vi "CCGetDICOMValuesFromFile.vi"(8 "error in (no error)":errorcluster, 11 "filename":string) -> (0 "error out":errorcluster, 3 "Array":string[](array[string]))   [LabVIEW 2013, in "ClearCanvasLibrary.lvlib"]
uses:
  Controls/Enum Variables.ctl
  C:/Users/Simon/SkyDrive/LabView/2013/DM2020/DICOM/ClearCanvasNewBuild/ClearCanvas.Dicom.dll
  ClearCanvasNewBuild/ClearCanvas.Dicom.dll
  ClearCanvasLibrary.lvlib
  main.lvlib
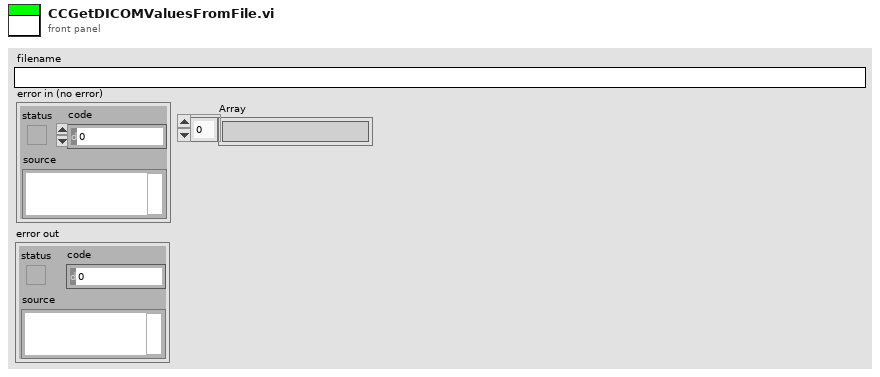
[diagram p1: front panel]
types:
  T1 = typedef "main.lvlib/Enum Variables.ctl" = enum16{"SetAcqFilter", "GetAcqFilter", "Set Filter", "Get Filter", "Set Height", "Get Height", "Set Blue Pressure", "Get Blue Pressure", "Set Red Pressure", "Get Red Pressure", "Init", "Reset Pressure", "Set Red Cursors", "Get Red Cursors", "Set Blue Cursors", "Get Blue Cursors", "Set Language", "Get Language", "Set Active Graphs", "Get ActiveGraphs", "Set Method", "Get Method", "Set Encryption", "Get Encryption", "Set ExcelVersion", "Get ExcelVersion", "Set itemTags", "Get itemTags", "Set Attributes", "Get Attributes", "Set DICOM Avail", "Get DICOM Avail", "Set DICOM Encode", "Get DICOM Encode", "Set JournalExport", "Get JournalExport", "Set Sequence", "Get Sequence", "Set DAQ Connected", "Get DAQ Connected", "Set Current Graph", "Get Current Graph", "Set General Settings", "Get Hyphenation", "Set Arm Calc Method", "Get Arm Calc Method", "Set Dicom Tags", "Get Dicom Tags"}
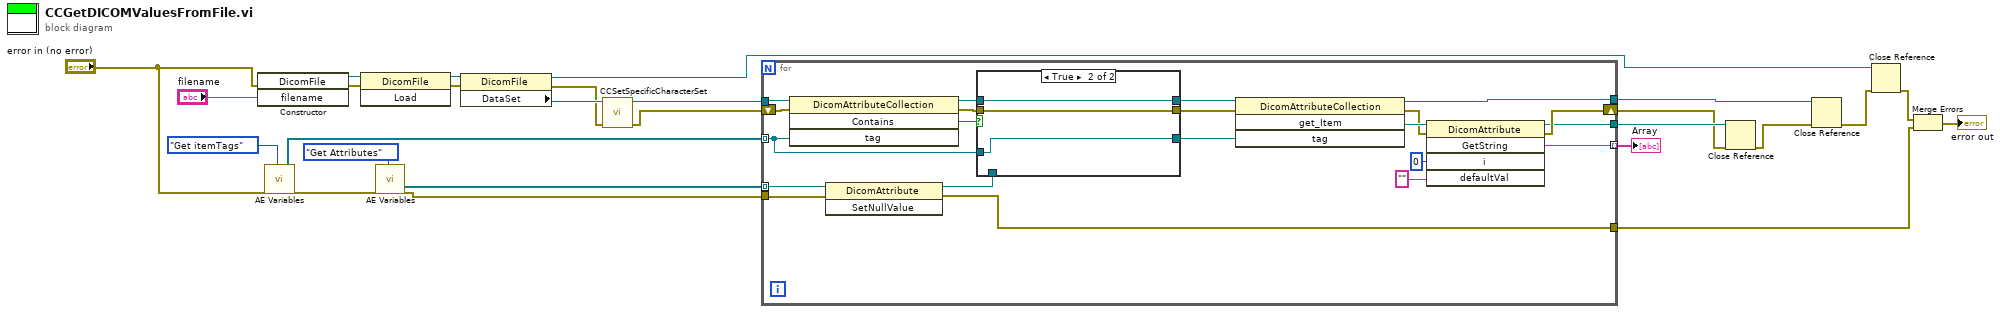
[diagram p0: block diagram]
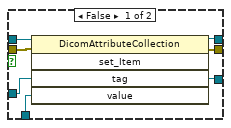
[diagram p2: hidden frame]
diagram:
  n1 = constructor class="DicomFile"(error in="error in (no error)", "filename"="filename") -> (reference out=w26:refnum<k24>, error out=w23:errorcluster)  [unwired: 2 in, 2 out]
  n2 = call "AE Variables.vi"("error in (no error)"="error in (no error)", "Action"=Enum_Variables."Get itemTags") -> ("itemTags .net"=w10:refnum<k24>[], "error out"=w9:errorcluster)  [unwired: 9 in, 7 out]
  n3 = invoke class="DicomFile" method="Load"(reference=w26, error in=w23) -> (reference out=w24:refnum<k24>, error out=w22:errorcluster)  [unwired: 1 in, 1 out]
  n4 = call "AE Variables.vi"("error in (no error)"=w9, "Action"=Enum_Variables."Get Attributes") -> (".net Array"=w7:refnum<k24>[], "error out"=w5:errorcluster)  [unwired: 9 in, 7 out]
  n5 = property class="DicomFile"(reference=w24, error in=w22) -> (reference out=w15:refnum<k24>, error out=w2:errorcluster, "DataSet"=w4:refnum<k24>)
  n6 = call "CCSetSpecificCharacterSet.vi"("error in (no error)"=w2, ".NET Refnum in"=w4) -> ("error out"=w1:errorcluster, ".NET Refnum out"=w3:refnum<k24>)  [unwired: 8 in]
  n7 = for {
    tunnel: w3 -> [w39]
    shift-right: [w42] -> w19
    shift-left: w1 -> [w38]
    tunnel: [w44] -> w21 mode=indexing
    tunnel: [w41] -> w20
    tunnel: [w40] -> w17
    tunnel: w10 -> [w33] mode=indexing
    tunnel: w7 -> [w30] mode=indexing
    tunnel: [w28] -> w6
    tunnel: w5 -> [w27]
    n8 = invoke class="DicomAttributeCollection" method="Contains"(reference=w39, error in=w38, "tag"=w33) -> (reference out=w36:refnum<k24>, error out=w34:errorcluster, "Contains"=w37:bool)  [unwired: 1 in, 1 out]
    n9 = invoke class="DicomAttribute" method="SetNullValue"(reference=w30, error in=w27) -> (reference out=w29:refnum<k24>, error out=w28:errorcluster)  [unwired: 1 in, 1 out]
    n10 = case shown="True" w37 {
      tunnel: w36 -> [w53 w56]
      tunnel: [w50 w56] -> w31
      tunnel: [w52 w55] -> w35
      tunnel: w34 -> [w51 w55]
      tunnel: w33 -> [w48 w54]
      tunnel: [w48 w54] -> w32
      tunnel: w29 -> [w49 _]
      frame False {
        n11 = invoke class="DicomAttributeCollection" method="set_Item"(reference=w53, error in=w51, "tag"=w48, "value"=w49) -> (reference out=w50:refnum<k24>, error out=w52:errorcluster)  [unwired: 1 in, 3 out]
      }
      frame True {
      }
    }
    n12 = invoke class="DicomAttributeCollection" method="get_Item"(reference=w31, error in=w35, "tag"=w32) -> (reference out=w40:refnum<k24>, error out=w43:errorcluster, "get_Item"=w47:refnum<k24>)  [unwired: 1 in, 1 out]
    n13 = invoke class="DicomAttribute" method="GetString"(reference=w47, error in=w43, "i"=0, "defaultVal"="") -> (reference out=w41:refnum<k24>, error out=w42:errorcluster, "GetString"=w44:string)  [unwired: 1 in, 2 out]
  }
  "Array" <- w21
  n14 = Close Reference(reference=w20, error in (no error)=w19) -> (error out=w18:errorcluster)
  n15 = Close Reference(reference=w17, error in (no error)=w18) -> (error out=w16:errorcluster)
  n16 = Close Reference(reference=w15, error in (no error)=w16) -> (error out=w13:errorcluster)
  n17 = Merge Errors(w13, w6) -> (→"error out":errorcluster)
